vi "3. Multiple Polynomial Configurations.vi"(8 "error in (no error)":errorcluster) -> (0 "error out":errorcluster)   [LabVIEW 2014]
uses:
  PolyA class/PolyA.lvclass
  <vilib>/LabVIEW Open Source Project/Configuration Manager/Manager/Decompose KVPs.vi
  <vilib>/LabVIEW Open Source Project/Configuration Manager/Manager/Write.vi
  <vilib>/JKI/JKI SMO/SMO/SMO.lvclass
  <vilib>/LabVIEW Open Source Project/Configuration Manager/Cache/ConfigManager.Cache.lvclass
  <vilib>/LabVIEW Open Source Project/Configuration Manager/Manager/ConfigManager.lvclass
  <vilib>/addons/_JKI Toolkits/Caraya/classes/Test/Test.lvclass
  <vilib>/addons/_JKI Toolkits/Caraya/classes/Assert/Assert.lvclass
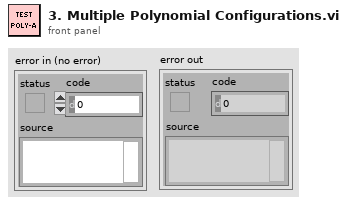
[diagram p1: front panel]
types:
  T1 = cluster{"Test Name":string, "Polynomials":dbl[], "Values":dbl[], "Results":dbl[]}[]
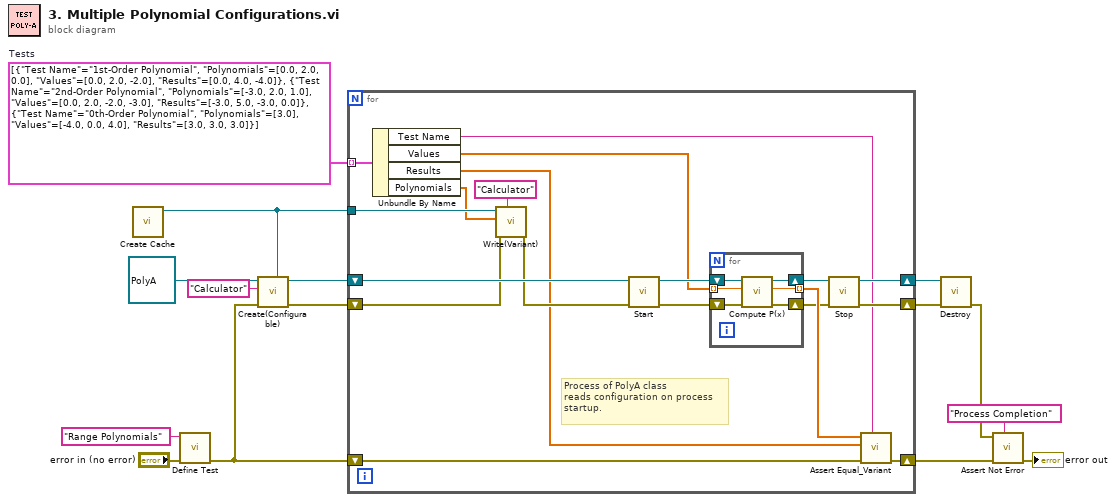
[diagram p0: block diagram]
diagram:
  w1 = T1 [{"Test Name"="1st-Order Polynomial", "Polynomials"=[0.0, 2.0, 0.0], "Values"=[0.0, 2.0, -2.0], "Results"=[0.0, 4.0, -4.0]}, {"Test Name"="2nd-Order Polynomial", "Polynomials"=[-3.0, 2.0, 1.0], "Values"=[0.0, 2.0, -2.0, -3.0], "Results"=[-3.0, 5.0, -3.0, 0.0]}, {"Test Name"="0th-Order Polynomial", "Polynomials"=[3.0], "Values"=[-4.0, 0.0, 4.0], "Results"=[3.0, 3.0, 3.0]}]  # Tests
  n1 = call <vilib>:"Create Cache.vi"() -> ("ConfigManager.Cache"=w2:refnum<class "ConfigManager.Cache.lvclass">)  [unwired: 11 in]
  n2 = call <vilib>:"Define Test.vi"("error in (no error)"="error in (no error)", "Label (VI Title)"="Range Polynomials") -> ("error out"=w8:errorcluster)  [unwired: 9 in]
  n3 = call <vilib>:"Create(Configurable).vi"("ConfigManager"=w2, "error in (no error)"=w8, "Subsystem Name (optional)"="Calculator", "SMO"=refnum<class "PolyA.lvclass"> refnum ("PolyA.lvclass")) -> ("error out"=w14:errorcluster, "SMO out"=w15:refnum<class "PolyA.lvclass">)  [unwired: 5 in, 1 out]
  n4 = for {
    shift-right: [w33] -> w13
    shift-left: w15 -> [w34]
    shift-right: [w32] -> w12
    shift-left: w14 -> [w23]
    shift-right: [w26] -> w4
    shift-left: w8 -> [w31]
    tunnel: w2 -> [w21]
    tunnel: w1 -> [w20] mode=indexing
    # "Process of PolyA class \nreads configuration on process\nstartup."
    n5 = Unbundle By Name(w20) -> ("Test Name"=w16:string, "Values"=w18:dbl[], "Results"=w17:dbl[], "Polynomials"=w19:dbl[])
    n6 = call <vilib>:"Write(Variant).vi"("Qualified Name"="Calculator" ("Subsystem Name (optional)"), "error in (no error)"=w23, "value"=w19, "ConfigManager in"=w21) -> ("error out"=w22:errorcluster)  [unwired: 5 in, 2 out]
    n7 = call <vilib>:"Start.vi"("error in (no error)"=w22, "SMO"=w34) -> ("error out"=w25:errorcluster, "SMO out"=w30:refnum<class "PolyA.lvclass">)  [unwired: 8 in]
    n8 = for {
      tunnel: [w39] -> w29 mode=indexing
      shift-right: [w38] -> w28
      shift-left: w30 -> [w40]
      shift-right: [w37] -> w27
      shift-left: w25 -> [w36]
      tunnel: w18 -> [w35] mode=indexing
      n9 = call "Compute P(x).vi"("error in (no error)"=w36, "x"=w35, "PolyA in"=w40) -> ("error out"=w37:errorcluster, "P(x)"=w39:dbl, "PolyA out"=w38:refnum<class "PolyA.lvclass">)  [unwired: 5 in, 1 out]
    }
    n10 = call <vilib>:"Stop.vi"("error in (no error)"=w27, "SMO"=w28) -> ("error out"=w32:errorcluster, "SMO out"=w33:refnum<class "PolyA.lvclass">)  [unwired: 8 in]
    n11 = call <vilib>:"Assert Equal_Variant.vi"("Label"=w16, "error in (no error)"=w31, "Y"=w17, "X"=w29) -> ("error out"=w26:errorcluster)  [unwired: 7 in]
  }
  n12 = call <vilib>:"Destroy.vi"("error in (no error)"=w12, "SMO"=w13) -> ("error out"=w7:errorcluster)  [unwired: 9 in]
  n13 = call <vilib>:"Assert Not Error.vi"("Label"="Process Completion" ("Label (VI Title)"), "error in (no error)"=w4, "Not Error?"=w7) -> ("error out"=→"error out":errorcluster)  [unwired: 8 in]
